vi "CTUD.vi"(6 "R":bool, 7 "Load":bool, 9 "DI":u32, 10 "-":bool, 11 "+":bool) -> (1 "DO":u32, 2 "ED":bool, 3 "EU":bool)   [LabVIEW 2019, in "Counter.lvlib"]
uses:
  Counter.lvlib
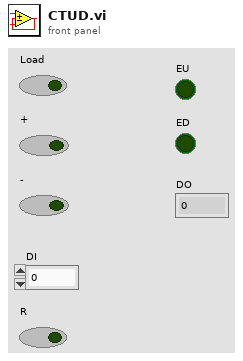
[diagram p1: front panel]
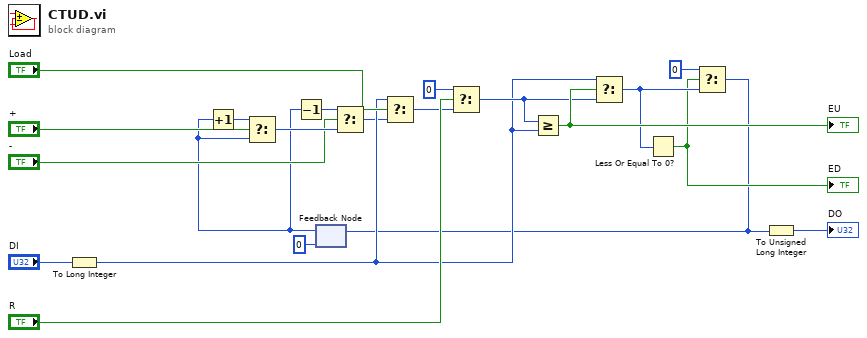
[diagram p0: block diagram]
diagram:
  n1 = To Long Integer(number="DI") -> (32bit integer=w10:i32)
  n2 = feedback #1(0) -> (w2:i32)
  n3 = Increment(x=w2) -> (x+1=w7:i32)
  n4 = Select(t=w7, s="+", f=w2) -> (s? t:f=w4:i32)
  n5 = Decrement(x=w2) -> (x-1=w5:i32)
  n6 = Select(t=w5, s="-", f=w4) -> (s? t:f=w1:i32)
  n7 = Select(t=w10, s="Load", f=w1) -> (s? t:f=w15:i32)
  n8 = Select(t=0, s="R", f=w15) -> (s? t:f=w17:i32)
  n9 = Greater Or Equal?(x=w17, y=w10) -> (x >= y?=w20:bool)
  "EU" <- w20
  n10 = Select(t=w10, s=w20, f=w17) -> (s? t:f=w14:i32)
  n11 = Less Or Equal To 0?(x=w14) -> (x <= 0?=w12:bool)
  "ED" <- w12
  n12 = Select(t=0, s=w12, f=w14) -> (s? t:f=w8:i32)
  n13 = feedback-in #1(w8) -> ()
  n14 = To Unsigned Long Integer(number=w8) -> (unsigned 32bit integer=→"DO":u32)
